vi "Get Filter Default State.vi"(8 "error in (no error)":errorcluster) -> (0 "error out":errorcluster, 3 "Filters Enabled By Default?":bool)   [LabVIEW 2017, in "Assert API Components.lvlib" / "Assert Display.lvlib" / "Filter Config Display.lvlib" / "Filter Config Display.lvclass"]
uses:
  Filter Config Display.lvclass
  <vilib>/Utility/config.llb/Read Key (Boolean).vi
  Assert API Components/Assert API Components.lvlib
  <vilib>/Utility/config.llb/NI_LVConfig.lvlib
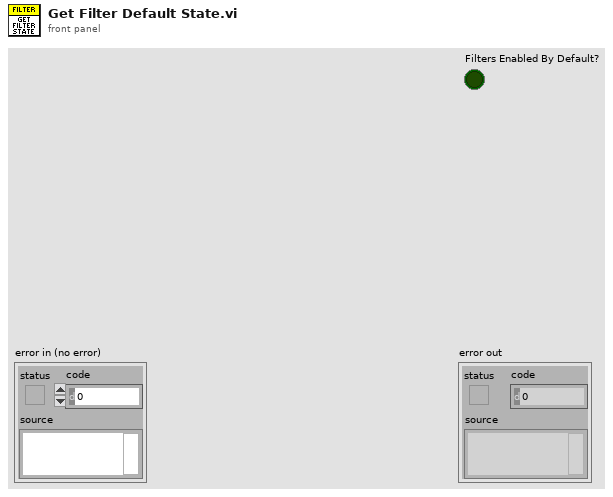
[diagram p1: front panel]
types:
  T1 = typedef "NI_LVConfig.lvlib/Config Data RefNum.ctl" = refnum<k1>
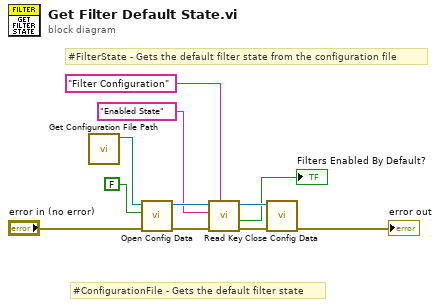
[diagram p0: block diagram]
diagram:
  # "#ConfigurationFile - Gets the default filter state"
  # "#FilterState - Gets the default filter state from the configuration file"
  n1 = call "Get Configuration File Path.vi"() -> ("Configuration File Path"=w5:path)  [unwired: 11 in]
  n2 = call <vilib>:"Open Config Data.vi"("error in (no error)"="error in (no error)", "create file if necessary (T)"=FALSE, "configuration file path"=w5) -> ("error out"=w10:errorcluster, "refnum"=w7:T1)  [unwired: 6 in, 1 out]
  n3 = call-poly <vilib>:"Read Key.vi"("section"="Filter Configuration", "error in (no error)"=w10, "key"="Enabled State", "refnum"=w7) -> ("error out"=w9:errorcluster, "value"=→"Filters Enabled By Default?":bool, "refnum out"=w6:T1)  [unwired: 4 in, 1 out]
  n4 = call <vilib>:"Close Config Data.vi"("error in (no error)"=w9, "refnum"=w6) -> ("error out"=→"error out":errorcluster)  [unwired: 8 in, 1 out]
